vi "PXDAC config-2 (SubVI).vi"(1 "Handle Out in":i64, 3 "first run?":bool=TRUE, 7 "calib (no out to AWG)":bool, 14 "config":T1={"BW [MHz]"=19.691598360655735, "Taod [us]"=29.10737386804657, "Nzf"=5, "Tpp [us]"=217.72315653298836, "Tdaod [us]"=1357.142857142857, "Tf2 [us]"=2395.569210866753, "Nv"=4.0, "ch1 range"=580.0, "ch2 range"=680.0, "wavel ratio"=0.871, "delay [us]"=-40.0, "calib(F)/monitor(T)"=FALSE}) -> (4 "Handle Out out":i64, 6 "Waveform":dbl[][](graph), 8 "size(s)":i32=1335296)   [LabVIEW 2024]
panel:
  in  "center freq [MHz] 2":dbl=150.0 format="%#_13g"
  in  "center freq [MHz]":dbl=150.0
  in  "base path":path=path "C:/Users/Mikamilab/Documents/lightsheet/LabVIEW3D/AWGfor3D/waveform.rd16"
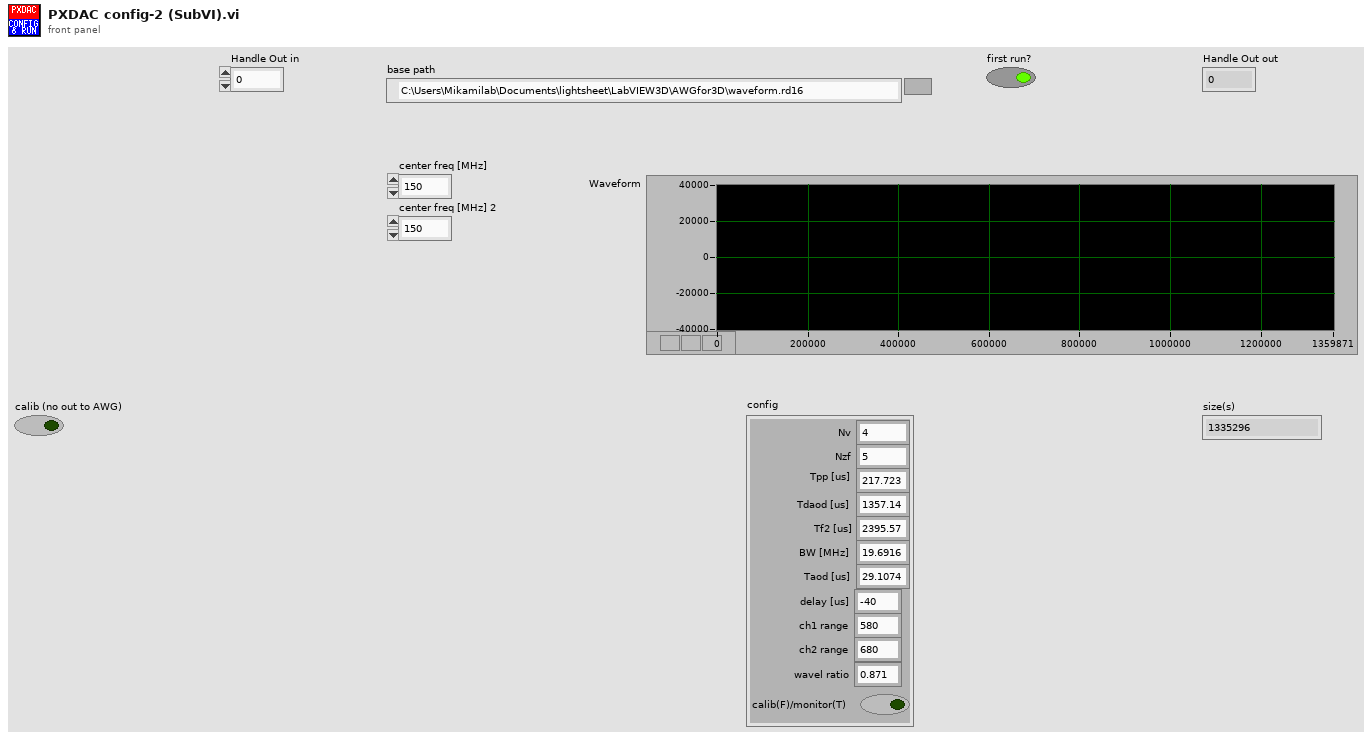
[diagram p1: front panel]
types:
  T1 = cluster{"BW [MHz]":dbl, "Taod [us]":dbl, "Nzf":i32, "Tpp [us]":dbl, "Tdaod [us]":dbl, "Tf2 [us]":dbl, "Nv":dbl, "ch1 range":dbl, "ch2 range":dbl, "wavel ratio":dbl, "delay [us]":dbl, "calib(F)/monitor(T)":bool}
  T2 = cluster{"BW [MHz]":dbl, "Taod [us]":dbl, "Nzf":i32, "Tpp [us]":dbl, "Tdaod [us]":dbl, "Tf2 [us]":dbl, "Nv":dbl}
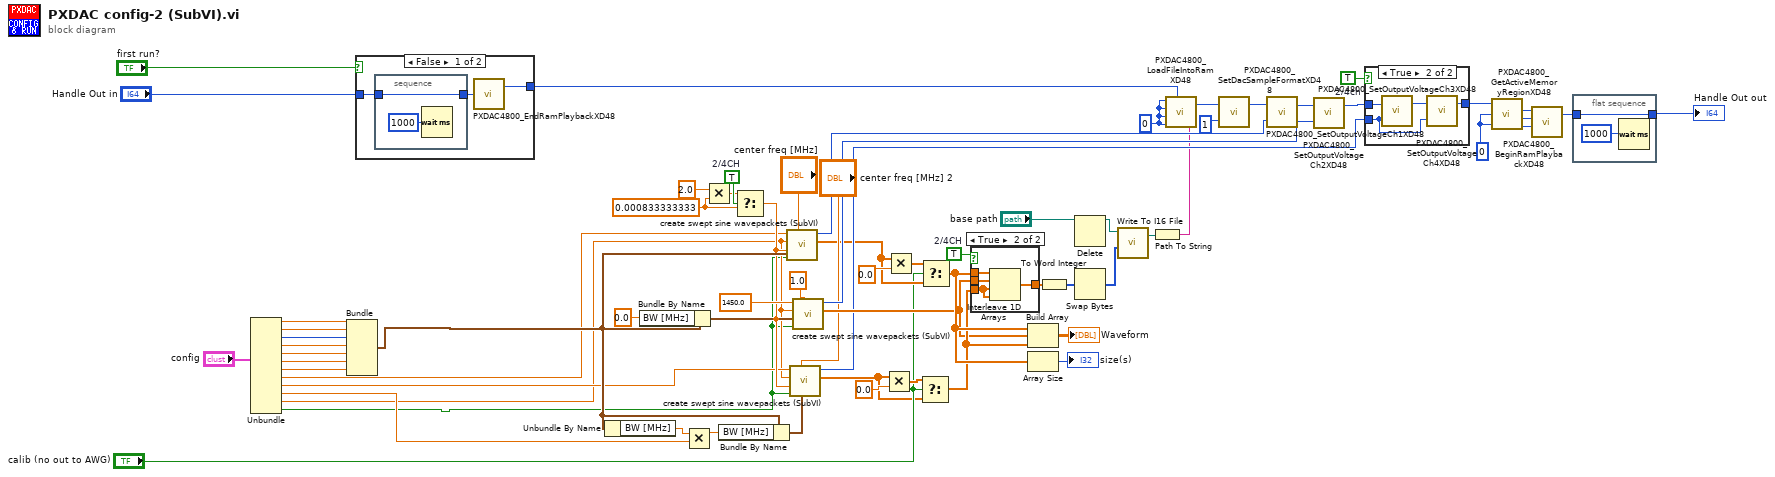
[diagram p0: block diagram]
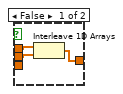
[diagram p4: hidden frame]
diagram:
  w64 = TRUE  # 2/4ch
  w61 = TRUE  # 2/4CH
  w63 = TRUE  # 2/4CH
  w53 = 0.000833333333 ("sampling period [us] in")
  w29 = u32 0 ("Offset")
  w23 = u32 0 ("src_length_bytes")
  n1 = Unbundle("config") -> ("BW [MHz]"=w1:dbl, "Taod [us]"=w2:dbl, "Nzf"=w3:i32, "Tpp [us]"=w4:dbl, "Tdaod [us]"=w5:dbl, "Tf2 [us]"=w6:dbl, "Nv"=w7:dbl, "ch1 range"=w13:dbl, "ch2 range"=w12:dbl, "wavel ratio"=w11:dbl, "delay [us]"=w10:dbl, "calib(F)/monitor(T)"=w9:bool)
  n2 = Bundle("BW [MHz]"=w1, "Taod [us]"=w2, "Nzf"=w3, "Tpp [us]"=w4, "Tdaod [us]"=w5, "Tf2 [us]"=w6, "Nv"=w7) -> (w37:T2)  [unwired: 1 in]
  n3 = case shown="False" "first run?" {
    tunnel: "Handle Out in" -> [w70 w74]
    tunnel: [w69 w74] -> w68
    frame False {
      n4 = stacked-sequence {
        tunnel: [w72] -> w71
        tunnel: w70 -> [w72]
        frame #0 {
          n5 = Wait (ms)(milliseconds to wait=1000) -> ()  [unwired: 1 out]
        }
      }
      n6 = call "PXDAC4800_EndRamPlaybackXD48.vi"("Handle"=w71) -> ("Handle out"=w69:i64)  [unwired: 1 out]
    }
    frame True {
    }
  }
  n7 = Unbundle By Name(w37) -> ("BW [MHz]"=w36:dbl)
  n8 = Bundle By Name(cluster=w37, "BW [MHz]"=0.0) -> (w38:T2)
  n9 = Multiply(x=w36, y=w11) -> (x*y=w35:dbl)
  n10 = Multiply(x=2.0 ("y"), y=w53) -> (x*y=w44:dbl)
  n11 = Bundle By Name(cluster=w37, "BW [MHz]"=w35) -> (w34:T2)
  n12 = Select(t=w44, s=w63, f=w53) -> (s? t:f=w33:dbl)
  n13 = call "create swept sine wavepackets (SubVI).vi"("Cluster"=w37, "center freq [MHz]"="center freq [MHz]", "calib(F)/monitor(T)"=w9, "sampling period [us] in"=w33, "delay [us]"=w10, "voltage range [470-1450mV]"=w13) -> ("Array"=w42:dbl[], "Numeric"=w58:u32)  [unwired: 4 in]
  n14 = call "create swept sine wavepackets (SubVI).vi"("Cluster"=w34, "center freq [MHz]"="center freq [MHz] 2", "calib(F)/monitor(T)"=w9, "sampling period [us] in"=w33, "delay [us]"=w10, "voltage range [470-1450mV]"=w12) -> ("Array"=w32:dbl[], "Numeric"=w55:u32)  [unwired: 4 in]
  n15 = call "create swept sine wavepackets (SubVI).vi"("Cluster"=w38, "center freq [MHz]"=1.0, "calib(F)/monitor(T)"=w9, "sampling period [us] in"=w33, "delay [us]"=w10, "voltage range [470-1450mV]"=1450.0) -> ("Array"=w56:dbl[], "Numeric"=w57:u32)  [unwired: 4 in]
  n16 = Multiply(x=w32, y=0.0) -> (x*y=w40:dbl[])
  n17 = Multiply(x=w42, y=0.0) -> (x*y=w41:dbl[])
  n18 = Select(t=w40, s="calib (no out to AWG)", f=w32) -> (s? t:f=w59:dbl[])
  n19 = Select(t=w41, s="calib (no out to AWG)", f=w42) -> (s? t:f=w60:dbl[])
  n20 = case shown="True" w61 {
    tunnel: w56 -> [w77 w80]
    tunnel: w60 -> [w76 w81]
    tunnel: [w75 w78] -> w16
    tunnel: w59 -> [_ w79]
    frame False {
      n21 = Interleave 1D Arrays(w76, w77) -> (w75:dbl[])
    }
    frame True {
      n22 = Interleave 1D Arrays(w81, w80, w79, w79) -> (w78:dbl[])
    }
  }
  n23 = Build Array(w60, w56, w59) -> (→"Waveform":dbl[][])
  n24 = Array Size(array=w60) -> (size(s)=→"size(s)":i32)
  n25 = To Word Integer(number=w16) -> (16bit integer=w14:i16[])
  n26 = Delete(path (use dialog)="base path") -> (deleted path=w17:path)  [unwired: 4 in, 2 out]
  n27 = Swap Bytes(anything=w14) -> (byte swapped=w15:i16[])
  n28 = call <vilib>:"Write To I16 File.vi"("1D array"=w15, "file path (dialog if empty)"=w17) -> ("new file path (Not A Path if cancelled)"=w24:path)  [unwired: 5 in]
  n29 = Path To String(path=w24) -> (string=w25:string)
  n30 = call "PXDAC4800_LoadFileIntoRamXD48.vi"("dst_offset_bytes"=w23, "Handle"=w68, "dst_length_bytes"=w23, "src_offset_bytes"=w23, "src_length_bytes"=w23, "File_Path"=w25) -> ("Handle Out"=w20:i64)  [unwired: 1 in, 1 out]
  n31 = call "PXDAC4800_SetDacSampleFormatXD48.vi"("Value"=u32 1, "Handle"=w20) -> ("Handle out"=w19:i64)  [unwired: 1 out]
  n32 = call "PXDAC4800_SetOutputVoltageCh1XD48.vi"("Value"=w58, "Handle"=w19) -> ("Handle out"=w21:i64)  [unwired: 1 out]
  n33 = call "PXDAC4800_SetOutputVoltageCh2XD48.vi"("Value"=w57, "Handle"=w21) -> ("Handle out"=w18:i64)  [unwired: 1 out]
  n34 = case shown="True" w64 {
    tunnel: w18 -> [w82 w86]
    tunnel: [w82 w84] -> w30
    tunnel: w55 -> [_ w83]
    frame False {
    }
    frame True {
      n35 = call "PXDAC4800_SetOutputVoltageCh3XD48.vi"("Value"=w83, "Handle"=w86) -> ("Handle out"=w85:i64)  [unwired: 1 out]
      n36 = call "PXDAC4800_SetOutputVoltageCh4XD48.vi"("Value"=w83, "Handle"=w85) -> ("Handle out"=w84:i64)  [unwired: 1 out]
    }
  }
  n37 = call "PXDAC4800_GetActiveMemoryRegionXD48.vi"("Handle"=w30, "Offset"=w29, "Length Byte"=w29) -> ("Handle out"=w28:i64, "Offset_bytes out"=w27:u32, "Playback_bytes out"=w26:u32)  [unwired: 1 out]
  n38 = call "PXDAC4800_BeginRamPlaybackXD48.vi"("ram length bytes"=w26, "ram offset bytes"=w27, "Handle"=w28) -> ("Handle Out"=w31:i64)  [unwired: 1 in, 1 out]
  n39 = flat-sequence {
    tunnel: w31 -> [w87]
    tunnel: [w87] -> w65
    frame #0 {
      n40 = Wait (ms)(milliseconds to wait=1000) -> ()  [unwired: 1 out]
    }
  }
  "Handle Out out" <- w65
